vi "set currentVI.vi"(8 "error in (no error)":errorcluster caption="错误输入（无错误）", 10 "CurrentVi*":refnum<vi>, 11 "PanelRootNode输入":refnum<class "PanelRootNode.lvclass">) -> (0 "error out":errorcluster caption="错误输出", 3 "PanelRootNode输出":refnum<class "PanelRootNode.lvclass">)   [LabVIEW 2013, in "PanelRootNode.lvclass"]
uses:
  PanelRootNode.lvclass
  PanelRootNode.lvclass/PanelRootNode.ctl
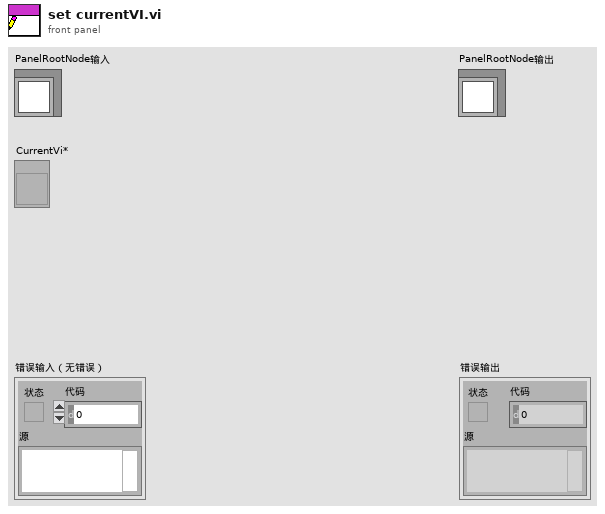
[diagram p1: front panel]
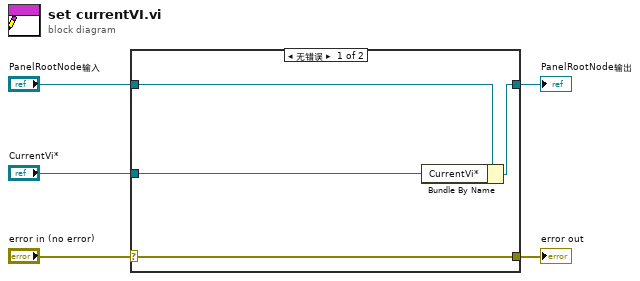
[diagram p0: block diagram]
diagram:
  n1 = case shown="无错误" "error in (no error)" {
    selector: "error in (no error)" -> [w9 w10]
    tunnel: [w9 w10] -> w4
    tunnel: [w7 w11] -> w2
    tunnel: "PanelRootNode输入" -> [w8 w11]
    tunnel: "CurrentVi*" -> [w6 _]
    frame No Error {
      n2 = Bundle By Name(cluster=w8, "CurrentVi*"=w6) -> (w7:refnum<class "PanelRootNode.lvclass">)
    }
    frame Error {
    }
  }
  "error out" <- w4
  "PanelRootNode输出" <- w2
